vi "Time string.vi"() -> ()   [LabVIEW 2012]
panel:
  out "double precision float 2":dbl
  out "double precision float":dbl
  out "concatenated string":string
  in  "Start time":timestamp
  in  "End time":timestamp
  in  "stop":bool
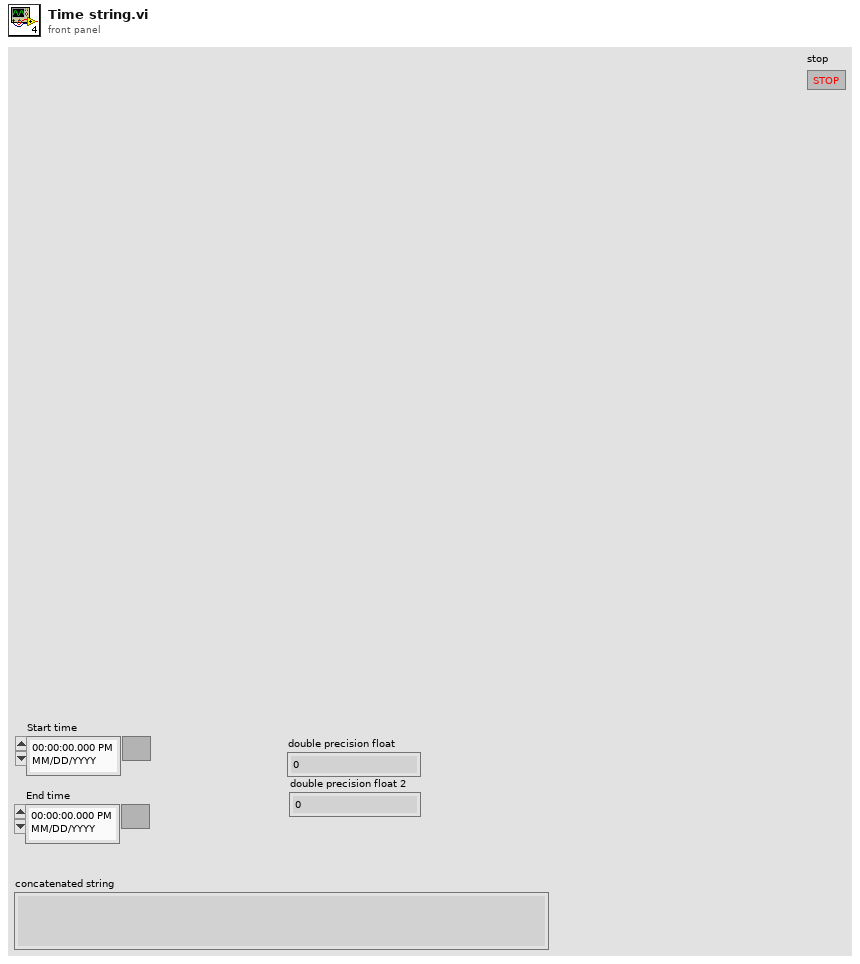
[diagram p1: front panel]
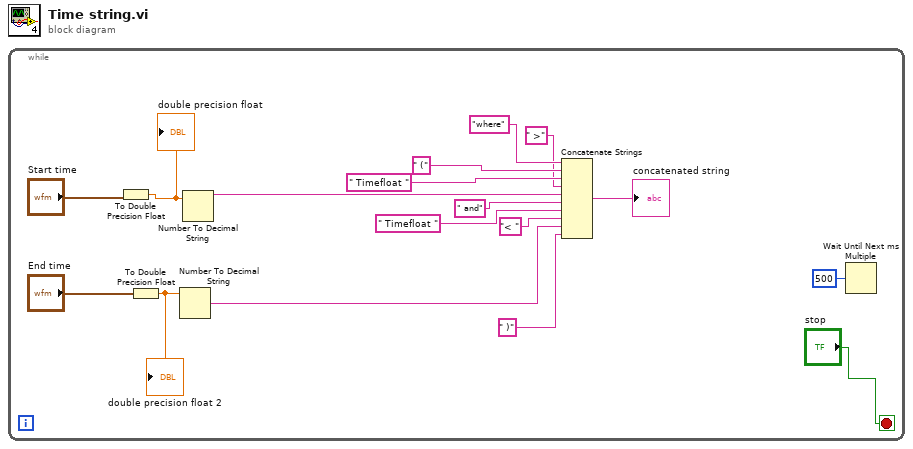
[diagram p0: block diagram]
diagram:
  n1 = while {
    stop <- "stop" stop-if-true
    n2 = To Double Precision Float(number="Start time") -> (double precision float=w9:dbl)
    "double precision float" <- w9
    n3 = To Double Precision Float(number="End time") -> (double precision float=w4:dbl)
    "double precision float 2" <- w4
    n4 = Number To Decimal String(number=w4) -> (decimal integer string=w3:string)  [unwired: 1 out]
    n5 = Number To Decimal String(number=w9) -> (decimal integer string=w8:string)  [unwired: 1 out]
    n6 = Concatenate Strings("where", " (", " Timefloat " ("string"), " >" ("string"), w8, " and", " Timefloat ", "< " ("string"), w3, " )") -> (→"concatenated string":string)
    n7 = Wait Until Next ms Multiple(millisecond multiple=u32 500) -> ()  [unwired: 1 out]
  }
